vi "MegaAnalysis5.vi"() -> ()   [LabVIEW 2016] (continued)
                      n495 = call <vilib>:"Check if File or Folder Exists.vi"("path"=w1236) -> ("file or folder exists?"=w1237:bool)  [unwired: 1 in, 9 out]
                      n496 = case shown="True" w1237 {
                        selector: w1237 -> [_ w1239]
                        tunnel: w1236 -> [_ w1238]
                        frame False {
                        }
                        frame True {
                          n497 = Delete(path (use dialog)=w1238, entire hierarchy (F)=w1239) -> ()  [unwired: 1 in, 5 out]
                        }
                      }
                    }
                    frame #1 {
                      n498 = Write to Text File(file (use dialog)=w1240, text=w1241) -> ()  [unwired: 1 in, 4 out]
                    }
                    frame #2 {
                      w1242 = TRUE
                      n499 = call "Write To Spreadsheet File2.vi"("transpose? (no:F)"=w1242, "format (%d)"=w1243, "append to file? (new file:F)"=w1242, "2D data"=w1245, "file path (dialog if empty)"=w1244) -> ()  [unwired: 3 in, 1 out]
                    }
                  }
                }
                n500 = global write "status.vi" "String"("saving import") -> ()
              }
            }
          }
          frame #19 {
            n501 = Or(x=w1254, y="?") -> (x .or. y?=w1255:bool)
            n502 = Reciprocal(x=w1258) -> (1/x=w1264:ext[])
            "sampling frequency" <- w1264
            n503 = Not Equal To 0?(x=w1258) -> (x != 0?=w1265:bool[])
            n504 = for {
              tunnel: w1255 -> [w1277]
              tunnel: "filter selection" -> [w1278]
              tunnel: w1265 -> [w1276] mode=indexing
              tunnel: w1264 -> [w1275] mode=indexing
              tunnel: w1263 -> [w1272]
              tunnel: "high cutoff freq: fh" -> [w1271]
              tunnel: "low cutoff freq: fl" -> [w1270]
              tunnel: "filter type" -> [w1269]
              tunnel: "order" -> [w1268]
              tunnel: w1257 -> [w1267]
              i -> [w1273]
              n505 = And(x=w1277, y=w1276) -> (x .and. y?=w1274:bool)
              n506 = case shown="True" w1274 {
                tunnel: w1278 -> [_ w1288]
                tunnel: w1275 -> [_ w1287]
                tunnel: w1273 -> [_ w1286]
                tunnel: w1272 -> [_ w1285]
                tunnel: w1271 -> [_ w1284]
                tunnel: w1270 -> [_ w1283]
                tunnel: w1269 -> [_ w1282]
                tunnel: w1268 -> [_ w1281]
                tunnel: w1267 -> [_ w1280]
                frame False {
                }
                frame True {
                  n507 = case shown="0, Default" w1288 {
                    tunnel: w1287 -> [_ w1294 w1309 w1324 w1340 w1354 w1370 _]
                    tunnel: w1286 -> [_ w1300 w1316 w1331 w1347 w1361 w1366 w1385]
                    tunnel: w1285 -> [_ w1299 w1315 w1330 w1346 w1360 w1376 w1387]
                    tunnel: w1284 -> [_ w1293 w1308 w1323 w1339 w1353 w1368 _]
                    tunnel: w1283 -> [_ w1292 w1307 w1322 w1338 w1352 w1369 _]
                    tunnel: w1282 -> [_ w1291 w1304 w1321 w1337 w1350 w1367 _]
                    tunnel: w1281 -> [_ w1290 w1306 w1319 w1336 w1351 _ _]
                    tunnel: w1280 -> [_ w1289 w1303 w1318 w1333 w1349 w1363 w1378]
                    frame 0, Default {
                    }
                    frame 1 {
                      w1301 = "dat2"
                      w1302 = "dat1"
                      n508 = call "readbinary.vi"(7:w1289, "base path"=w1299, "file index"=w1300, "data column"=w1302) -> ("data"=w1297:ext[])  [unwired: 7 out]
                      n509 = call "readbinary.vi"(7:w1289, "base path"=w1299, "file index"=w1300, "data column"=w1301) -> ("data"=w1298:ext[])  [unwired: 7 out]
                      n510 = call-poly <vilib>:"Butterworth Filter.vi"("order"=w1290, "filter type"=w1291, "low cutoff freq: fl"=w1292, "high cutoff freq: fh"=w1293, "sampling freq: fs"=w1294, "X"=w1297) -> ("Filtered X"=w1296:dbl[])  [unwired: 1 in, 2 out]
                      n511 = call-poly <vilib>:"Butterworth Filter.vi"("order"=w1290, "filter type"=w1291, "low cutoff freq: fl"=w1292, "high cutoff freq: fh"=w1293, "sampling freq: fs"=w1294, "X"=w1298) -> ("Filtered X"=w1295:dbl[])  [unwired: 1 in, 2 out]
                      n512 = call "writebinary.vi"(7:w1289, "base path"=w1299, "file index"=w1300, "data column"=w1302, "data"=w1296) -> ()  [unwired: 7 out]
                      n513 = call "writebinary.vi"(7:w1289, "base path"=w1299, "file index"=w1300, "data column"=w1301, "data"=w1295) -> ()  [unwired: 7 out]
                    }
                    frame 2 {
                      w1317 = "dat2"
                      w1313 = "dat1"
                      n514 = call "readbinary.vi"(7:w1303, "base path"=w1315, "file index"=w1316, "data column"=w1313) -> ("data"=w1312:ext[])  [unwired: 7 out]
                      n515 = call "readbinary.vi"(7:w1303, "base path"=w1315, "file index"=w1316, "data column"=w1317) -> ("data"=w1314:ext[])  [unwired: 7 out]
                      n516 = call-poly <vilib>:"Chebyshev Filter.vi"("order"=w1306, "ripple(dB)"="ripple(dB)", "filter type"=w1304, "low cutoff freq: fl"=w1307, "high cutoff freq: fh"=w1308, "sampling freq: fs"=w1309, "X"=w1314) -> ("Filtered X"=w1310:dbl[])  [unwired: 1 in, 3 out]
                      n517 = call-poly <vilib>:"Chebyshev Filter.vi"("order"=w1306, "ripple(dB)"="ripple(dB)", "filter type"=w1304, "low cutoff freq: fl"=w1307, "high cutoff freq: fh"=w1308, "sampling freq: fs"=w1309, "X"=w1312) -> ("Filtered X"=w1311:dbl[])  [unwired: 1 in, 3 out]
                      n518 = call "writebinary.vi"(7:w1303, "base path"=w1315, "file index"=w1316, "data column"=w1313, "data"=w1311) -> ()  [unwired: 7 out]
                      n519 = call "writebinary.vi"(7:w1303, "base path"=w1315, "file index"=w1316, "data column"=w1317, "data"=w1310) -> ()  [unwired: 7 out]
                    }
                    frame 3 {
                      w1332 = "dat2"
                      w1329 = "dat1"
                      n520 = call "readbinary.vi"(7:w1318, "base path"=w1330, "file index"=w1331, "data column"=w1329) -> ("data"=w1326:ext[])  [unwired: 7 out]
                      n521 = call "readbinary.vi"(7:w1318, "base path"=w1330, "file index"=w1331, "data column"=w1332) -> ("data"=w1328:ext[])  [unwired: 7 out]
                      n522 = call-poly <vilib>:"Inverse Chebyshev Filter.vi"("order"=w1319, "attenuation (dB)"="attenuation (dB)", "filter type"=w1321, "low cutoff freq: fl"=w1322, "high cutoff freq: fh"=w1323, "sampling freq: fs"=w1324, "X"=w1328) -> ("Filtered X"=w1327:dbl[])  [unwired: 1 in, 3 out]
                      n523 = call-poly <vilib>:"Inverse Chebyshev Filter.vi"("order"=w1319, "attenuation (dB)"="attenuation (dB)", "filter type"=w1321, "low cutoff freq: fl"=w1322, "high cutoff freq: fh"=w1323, "sampling freq: fs"=w1324, "X"=w1326) -> ("Filtered X"=w1325:dbl[])  [unwired: 1 in, 3 out]
                      n524 = call "writebinary.vi"(7:w1318, "base path"=w1330, "file index"=w1331, "data column"=w1329, "data"=w1325) -> ()  [unwired: 7 out]
                      n525 = call "writebinary.vi"(7:w1318, "base path"=w1330, "file index"=w1331, "data column"=w1332, "data"=w1327) -> ()  [unwired: 7 out]
                    }
                    frame 4 {
                      w1348 = "dat2"
                      w1345 = "dat1"
                      n526 = call "readbinary.vi"(7:w1333, "base path"=w1346, "file index"=w1347, "data column"=w1345) -> ("data"=w1343:ext[])  [unwired: 7 out]
                      n527 = call "readbinary.vi"(7:w1333, "base path"=w1346, "file index"=w1347, "data column"=w1348) -> ("data"=w1344:ext[])  [unwired: 7 out]
                      n528 = call-poly <vilib>:"Elliptic Filter.vi"("order"=w1336, "filter type"=w1337, "stopband attenuation (dB)"="stopband attenuation (dB)", "passband ripple (dB)"="passband ripple (dB)", "low cutoff freq: fl"=w1338, "high cutoff freq: fh"=w1339, "sampling freq: fs"=w1340, "X"=w1343) -> ("Filtered X"=w1342:dbl[])  [unwired: 1 in, 2 out]
                      n529 = call-poly <vilib>:"Elliptic Filter.vi"("order"=w1336, "filter type"=w1337, "stopband attenuation (dB)"="stopband attenuation (dB)", "passband ripple (dB)"="passband ripple (dB)", "low cutoff freq: fl"=w1338, "high cutoff freq: fh"=w1339, "sampling freq: fs"=w1340, "X"=w1344) -> ("Filtered X"=w1341:dbl[])  [unwired: 1 in, 2 out]
                      n530 = call "writebinary.vi"(7:w1333, "base path"=w1346, "file index"=w1347, "data column"=w1345, "data"=w1342) -> ()  [unwired: 7 out]
                      n531 = call "writebinary.vi"(7:w1333, "base path"=w1346, "file index"=w1347, "data column"=w1348, "data"=w1341) -> ()  [unwired: 7 out]
                    }
                    frame 5 {
                      w1362 = "dat2"
                      w1359 = "dat1"
                      n532 = call "readbinary.vi"(7:w1349, "base path"=w1360, "file index"=w1361, "data column"=w1359) -> ("data"=w1357:ext[])  [unwired: 7 out]
                      n533 = call "readbinary.vi"(7:w1349, "base path"=w1360, "file index"=w1361, "data column"=w1362) -> ("data"=w1358:ext[])  [unwired: 7 out]
                      n534 = call-poly <vilib>:"Bessel Filter.vi"("order"=w1351, "filter type"=w1350, "low cutoff freq: fl"=w1352, "high cutoff freq: fh"=w1353, "sampling freq: fs"=w1354, "X"=w1357) -> ("Filtered X"=w1356:dbl[])  [unwired: 1 in, 2 out]
                      n535 = call-poly <vilib>:"Bessel Filter.vi"("order"=w1351, "filter type"=w1350, "low cutoff freq: fl"=w1352, "high cutoff freq: fh"=w1353, "sampling freq: fs"=w1354, "X"=w1358) -> ("Filtered X"=w1355:dbl[])  [unwired: 1 in, 2 out]
                      n536 = call "writebinary.vi"(7:w1349, "base path"=w1360, "file index"=w1361, "data column"=w1359, "data"=w1356) -> ()  [unwired: 7 out]
                      n537 = call "writebinary.vi"(7:w1349, "base path"=w1360, "file index"=w1361, "data column"=w1362, "data"=w1355) -> ()  [unwired: 7 out]
                    }
                    frame 6 {
                      w1377 = "dat2"
                      w1375 = "dat1"
                      n538 = call "readbinary.vi"(7:w1363, "base path"=w1376, "file index"=w1366, "data column"=w1375) -> ("data"=w1373:ext[])  [unwired: 7 out]
                      n539 = call "readbinary.vi"(7:w1363, "base path"=w1376, "file index"=w1366, "data column"=w1377) -> ("data"=w1374:ext[])  [unwired: 7 out]
                      n540 = call <vilib>:"FIR Windowed Filter (obs).vi"("sampling freq: fs"=w1370, "X"=w1373, "filter type"=w1367, "low cutoff freq: fl"=w1369, "high cutoff freq: fh"=w1368, "taps"="taps", "window"="window") -> ("Filtered X"=w1372:dbl[])  [unwired: 8 out]
                      n541 = call <vilib>:"FIR Windowed Filter (obs).vi"("sampling freq: fs"=w1370, "X"=w1374, "filter type"=w1367, "low cutoff freq: fl"=w1369, "high cutoff freq: fh"=w1368, "taps"="taps", "window"="window") -> ("Filtered X"=w1371:dbl[])  [unwired: 8 out]
                      n542 = call "writebinary.vi"(7:w1363, "base path"=w1376, "file index"=w1366, "data column"=w1375, "data"=w1372) -> ()  [unwired: 7 out]
                      n543 = call "writebinary.vi"(7:w1363, "base path"=w1376, "file index"=w1366, "data column"=w1377, "data"=w1371) -> ()  [unwired: 7 out]
                    }
                    frame 7 {
                      w1388 = "dat2"
                      w1386 = "dat1"
                      n544 = call "readbinary.vi"(7:w1378, "base path"=w1387, "file index"=w1385, "data column"=w1386) -> ("data"=w1383:ext[])  [unwired: 7 out]
                      n545 = call "readbinary.vi"(7:w1378, "base path"=w1387, "file index"=w1385, "data column"=w1388) -> ("data"=w1384:ext[])  [unwired: 7 out]
                      n546 = call <vilib>:"Median Filter.vi"("right rank"="right rank", "left rank"="left rank", "X"=w1383) -> ("Filtered X"=w1382:dbl[])  [unwired: 8 out]
                      n547 = call <vilib>:"Median Filter.vi"("right rank"="right rank", "left rank"="left rank", "X"=w1384) -> ("Filtered X"=w1381:dbl[])  [unwired: 8 out]
                      n548 = call "writebinary.vi"(7:w1378, "base path"=w1387, "file index"=w1385, "data column"=w1386, "data"=w1382) -> ()  [unwired: 7 out]
                      n549 = call "writebinary.vi"(7:w1378, "base path"=w1387, "file index"=w1385, "data column"=w1388, "data"=w1381) -> ()  [unwired: 7 out]
                    }
                  }
                  n550 = global write "status.vi" "String"("filtering") -> ()
                }
              }
            }
          }
          frame #20 {
            n551 = case shown="True" w1392 {
              tunnel: w1391 -> [_ w1395]
              tunnel: w1390 -> [_ w1394]
              tunnel: w1389 -> [_ w1393]
              frame False {
              }
              frame True {
                n552 = Path To String(path=w1394) -> (string=w1400:string[])
                n553 = Build Path(base path=w1395, name or relative path="files") -> (appended path=w1397:path)
                n554 = call-poly <vilib>:"Write To Spreadsheet File.vi"("1D data"=w1393, "file path (dialog if empty)"=w1397) -> ()  [unwired: 4 in, 3 out]
                n555 = Build Path(base path=w1395, name or relative path="paths") -> (appended path=w1399:path)
                n556 = call-poly <vilib>:"Write To Spreadsheet File.vi"("1D data"=w1400, "file path (dialog if empty)"=w1399) -> ()  [unwired: 4 in, 3 out]
              }
            }
          }
        }
      }
      frame #5 {
        # "select frame"
        # "old"
        # "both"
        # "rising"
        # "falling"
        # "c"
        # "p"
        n557 = Equal?(x=w1416, y=2) -> (x = y?=w1412:bool)
        n558 = Equal?(x="?", y=5) -> (x = y?=w1411:bool)
        n559 = And(x=w1412, y=w1411) -> (x .and. y?=w1410:bool)
        n560 = Or(x="?", y=w1403) -> (x .or. y?=w1405:bool)
        n561 = stacked-sequence {
          seq-local: [w1435 _ _ _ _ _ _ _ _ _] -> [_ _ _ _ _ w2421 w2652 w3048 w3122 _]
          seq-local: [w1434 _ _ _ _ _ _ _ _ _] -> [_ _ _ _ _ w2420 w2651 w3049 w3113 _]
          seq-local: [w1433 _ _ _ _ _ _ _ _ _] -> [_ w1485 w2161 _ _ w2422 _ _ _ _]
          seq-local: [w1422 _ _ _ _ _ _ _ _ _] -> [_ w1484 _ _ _ _ _ _ _ _]
          tunnel: w1405 -> [_ w1486 w2160 w2233 w2389 w2424 w2654 _ _ _]
          tunnel: w1417 -> [w1418 w1489 w2162 w2232 w2388 w2423 w2653 w3050 w3112 w3202]
          tunnel: w1410 -> [_ _ _ _ _ _ _ w3051 _ _]
          tunnel: "?" -> [_ _ _ _ _ _ _ _ w3123 _]
          tunnel: w1408 -> [_ w1483 _ _ _ _ _ _ w3111 _]
          tunnel: w1407 -> [w1419 w1482 w2159 w2231 w2387 w2419 w2650 w3046 _ _]
          tunnel: w1406 -> [w1420 _ _ _ _ _ _ _ _ _]
          tunnel: w1402 -> [_ _ _ _ _ _ _ _ w3110 _]
          tunnel: [_ _ _ _ _ _ _ _ w3109 _] -> w1401
          frame #0 {
            n562 = Build Array("indr", "timr", "bdtr", "bclr", "datr") -> (w1435:string[])
            n563 = Build Array("indf", "timf", "bdtf", "bclf", "datf") -> (w1434:string[])
            n564 = Build Array("indx", "time", "bdot", "bcol", "dat1", "dat2") -> (w1422:string[])
            n565 = Build Array("indt", "timt", "bdtt", "bclt", "dt1t", "dt2t") -> (w1433:string[])
            n566 = Build Path(base path=w1418, name or relative path="files") -> (appended path=w1430:path)
            n567 = Build Array (concatenate)(w1435, w1434, w1433) -> (w1432:string[])
            n568 = call-poly <vilib>:"Read From Spreadsheet File.vi"("file path (dialog if empty)"=w1430) -> ("first row"=w1429:string[])  [unwired: 3 in, 7 out]
            n569 = stacked-sequence {
              tunnel: w1432 -> [w1453 w1465]
              tunnel: w1418 -> [w1452 w1464]
              tunnel: w1429 -> [w1451 w1463]
              tunnel: w1420 -> [_ w1461]
              tunnel: w1419 -> [_ w1460]
              frame #0 {
                n570 = for {
                  tunnel: w1453 -> [w1456]
                  tunnel: w1452 -> [w1455]
                  tunnel: w1451 -> [_] mode=indexing
                  i -> [w1454]
                  n571 = for {
                    tunnel: w1456 -> [w1459] mode=indexing
                    tunnel: w1455 -> [w1458]
                    tunnel: w1454 -> [w1457]
                    n572 = call "createemptybinary.vi"("base path"=w1458, "file index"=w1457, "data column"=w1459) -> ()  [unwired: 9 out]
                  }
                }
              }
              frame #1 {
                n573 = Equal?(x=w1461, y=w1460) -> (x = y?=w1462:bool)
                n574 = case shown="False" w1462 {
                  tunnel: w1463 -> [w1470 _]
                  tunnel: w1465 -> [w1469 _]
                  tunnel: w1461 -> [w1468 _]
                  tunnel: w1460 -> [w1467 _]
                  tunnel: w1464 -> [w1466 _]
                  frame False {
                    n575 = for {
                      tunnel: w1470 -> [_] mode=indexing
                      tunnel: w1469 -> [w1475]
                      tunnel: w1466 -> [w1473]
                      tunnel: w1468 -> [w1472]
                      tunnel: w1467 -> [w1471]
                      i -> [w1474]
                      n576 = for {
                        tunnel: w1475 -> [w1478] mode=indexing
                        tunnel: w1474 -> [w1477]
                        tunnel: w1473 -> [w1476]
                        tunnel: w1472 -> [w1481]
                        tunnel: w1471 -> [w1479]
                        n577 = call "readbinary.vi"(7:w1481, "base path"=w1476, "file index"=w1477, "data column"=w1478) -> ("data"=w1480:ext[])  [unwired: 7 out]
                        n578 = call "writebinary.vi"(7:w1479, "base path"=w1476, "file index"=w1477, "data column"=w1478, "data"=w1480) -> ()  [unwired: 7 out]
                      }
                    }
                  }
                  frame True {
                  }
                }
              }
            }
          }
          frame #1 {
            n579 = case shown="False" w1486 {
              tunnel: "?" -> [_ w1501]
              tunnel: "reference option" -> [_ w1500]
              tunnel: w1489 -> [_ w1499]
              tunnel: "file name options" -> [_ w1498]
              tunnel: "?" -> [_ w1497]
              tunnel: w1485 -> [_ w1496]
              tunnel: w1484 -> [_ w1495]
              tunnel: w1483 -> [_ w1494]
              tunnel: w1482 -> [_ w1493]
              frame False {
              }
              frame True {
                n580 = case shown="False" w1501 {
                  tunnel: w1500 -> [_ w1536]
                  tunnel: w1499 -> [w1505 w1535]
                  tunnel: w1498 -> [_ w1534]
                  tunnel: w1497 -> [_ w1533]
                  tunnel: w1496 -> [w1506 _]
                  tunnel: w1495 -> [w1504 _]
                  tunnel: w1494 -> [w1503 w1532]
                  tunnel: w1493 -> [w1502 w1531]
                  frame False {
                    n581 = Build Path(base path=w1505, name or relative path="paths") -> (appended path=w1513:path)
                    n582 = Build Path(base path=w1505, name or relative path="files") -> (appended path=w1514:path)
                    n583 = call-poly <vilib>:"Read From Spreadsheet File.vi"("file path (dialog if empty)"=w1513) -> ("first row"=w1507:string[])  [unwired: 3 in, 7 out]
                    n584 = call-poly <vilib>:"Read From Spreadsheet File.vi"("file path (dialog if empty)"=w1514) -> ("first row"=w1508:string[])  [unwired: 3 in, 7 out]
                    n585 = Build Path(base path=w1505, name or relative path="files2") -> (appended path=w1510:path)
                    n586 = Build Path(base path=w1505, name or relative path="paths2") -> (appended path=w1509:path)
                    n587 = for {
                      tunnel: w1507 -> [_] mode=indexing
                      tunnel: w1506 -> [w1522]
                      tunnel: w1505 -> [w1521]
                      tunnel: w1504 -> [w1520]
                      tunnel: w1503 -> [w1518]
                      tunnel: w1502 -> [w1517]
                      i -> [w1519]
                      n588 = for {
                        tunnel: w1522 -> [w1527] mode=indexing
                        tunnel: w1519 -> [w1530]
                        tunnel: w1521 -> [w1525]
                        tunnel: w1520 -> [w1529] mode=indexing
                        tunnel: w1519 -> [w1526]
                        tunnel: w1518 -> [w1524]
                        tunnel: w1517 -> [w1523]
                        n589 = call "readbinary.vi"(7:w1524, "base path"=w1525, "file index"=w1530, "data column"=w1529) -> ("data"=w1528:ext[])  [unwired: 7 out]
                        n590 = call "writebinary.vi"(7:w1523, "base path"=w1525, "file index"=w1526, "data column"=w1527, "data"=w1528) -> ()  [unwired: 7 out]
                      }
                    }
                    n591 = call-poly <vilib>:"Write To Spreadsheet File.vi"("1D data"=w1508, "file path (dialog if empty)"=w1510) -> ()  [unwired: 4 in, 3 out]
                    n592 = call-poly <vilib>:"Write To Spreadsheet File.vi"("1D data"=w1507, "file path (dialog if empty)"=w1509) -> ()  [unwired: 4 in, 3 out]
                  }
                  frame True {
                    n593 = case shown="1" w1536 {
                      tunnel: w1535 -> [w1541 w1701 w1851 w2011]
                      tunnel: w1534 -> [w1540 w1700 w1850 w2010]
                      tunnel: w1533 -> [w1539 w1699 w1849 w2009]
                      tunnel: w1532 -> [w1538 w1698 w1848 w2008]
                      tunnel: w1531 -> [w1537 w1697 w1847 w2007]
                      frame 0, Default {
                        n594 = stacked-sequence {
                          seq-local: [w1544 _ _ _ _ _ _ _] -> [_ w1557 w1576 w1595 w1616 w1637 w1653 w1674]
                          seq-local: [w1542 _ _ _ _ _ _ _] -> [_ _ _ _ _ _ _ w1671]
                          tunnel: w1541 -> [w1548 w1553 w1572 w1591 w1612 w1633 w1649 w1663]
                          tunnel: w1540 -> [_ _ _ _ _ _ _ w1673]
                          tunnel: w1539 -> [_ _ _ _ _ _ _ w1672]
                          tunnel: w1538 -> [_ w1552 w1571 w1590 w1611 w1632 w1648 _]
                          tunnel: w1537 -> [_ w1551 w1570 w1589 w1610 w1631 w1647 _]
                          frame #0 {
                            w1546 = "%s"
                            n595 = Build Path(base path=w1548, name or relative path="files") -> (appended path=w1549:path)
                            n596 = call-poly <vilib>:"Read From Spreadsheet File.vi"("format (%s)"=w1546, "file path (dialog if empty)"=w1549) -> ("first row"=w1544:string[])  [unwired: 2 in, 7 out]
                            n597 = Build Path(base path=w1548, name or relative path="paths") -> (appended path=w1545:path)
                            n598 = call-poly <vilib>:"Read From Spreadsheet File.vi"("format (%s)"=w1546, "file path (dialog if empty)"=w1545) -> ("first row"=w1543:string[])  [unwired: 2 in, 7 out]
                            n599 = String To Path(string=w1543) -> (path=w1542:path[])
                          }
                          frame #1 {
                            n600 = Array Size(array=w1557) -> (size(s)=w1556:i32)
                            n601 = Divide(x=w1556, y=2) -> (x/y=w1554:dbl)
                            n602 = for {
                              N: w1554 -> [_]
                              tunnel: w1553 -> [w1561]
                              tunnel: w1552 -> [w1559]
                              tunnel: w1551 -> [w1558]
                              i -> [w1562]
                              w1564 = "dat1"
                              n603 = Multiply(x=2, y=w1562) -> (x*y=w1568:i32)
                              n604 = Increment(x=w1568) -> (x+1=w1567:i32)
                              n605 = call "readbinary.vi"(7:w1559, "base path"=w1561, "file index"=w1568, "data column"=w1564) -> ("data"=w1566:ext[])  [unwired: 7 out]
                              n606 = call "readbinary.vi"(7:w1559, "base path"=w1561, "file index"=w1567, "data column"=w1564) -> ("data"=w1565:ext[])  [unwired: 7 out]
                              n607 = Subtract(x=w1566, y=w1565) -> (x-y=w1563:ext[])
                              n608 = call "writebinary.vi"(7:w1558, "base path"=w1561, "file index"=w1562, "data column"="dt1t", "data"=w1563) -> ()  [unwired: 7 out]
                            }
                          }
                          frame #2 {
                            n609 = Array Size(array=w1576) -> (size(s)=w1575:i32)
                            n610 = Divide(x=w1575, y=2) -> (x/y=w1573:dbl)
                            n611 = for {
                              N: w1573 -> [_]
                              tunnel: w1572 -> [w1580]
                              tunnel: w1571 -> [w1578]
                              tunnel: w1570 -> [w1577]
                              i -> [w1581]
                              w1583 = "dat2"
                              n612 = Multiply(x=2, y=w1581) -> (x*y=w1587:i32)
                              n613 = Increment(x=w1587) -> (x+1=w1586:i32)
                              n614 = call "readbinary.vi"(7:w1578, "base path"=w1580, "file index"=w1587, "data column"=w1583) -> ("data"=w1585:ext[])  [unwired: 7 out]
                              n615 = call "readbinary.vi"(7:w1578, "base path"=w1580, "file index"=w1586, "data column"=w1583) -> ("data"=w1584:ext[])  [unwired: 7 out]
                              n616 = Subtract(x=w1585, y=w1584) -> (x-y=w1582:ext[])
                              n617 = call "writebinary.vi"(7:w1577, "base path"=w1580, "file index"=w1581, "data column"="dt2t", "data"=w1582) -> ()  [unwired: 7 out]
                            }
                          }
                          frame #3 {
                            n618 = Array Size(array=w1595) -> (size(s)=w1594:i32)
                            n619 = Divide(x=w1594, y=2) -> (x/y=w1592:dbl)
                            n620 = for {
                              N: w1592 -> [_]
                              tunnel: w1591 -> [w1604]
                              tunnel: w1590 -> [w1597]
                              tunnel: w1589 -> [w1596]
                              i -> [w1605]
                              w1606 = "bcol"
                              n621 = Multiply(x=2, y=w1605) -> (x*y=w1608:i32)
                              n622 = Increment(x=w1608) -> (x+1=w1607:i32)
                              n623 = call "readbinary.vi"(7:w1597, "base path"=w1604, "file index"=w1608, "data column"=w1606) -> ("data"=w1601:ext[])  [unwired: 7 out]
                              n624 = call "readbinary.vi"(7:w1597, "base path"=w1604, "file index"=w1607, "data column"=w1606) -> ("data"=w1600:ext[])  [unwired: 7 out]
                              n625 = Add(x=w1601, y=w1600) -> (x+y=w1603:ext[])
                              n626 = Divide(x=w1603, y=2) -> (x/y=w1599:ext[])
                              n627 = call "writebinary.vi"(7:w1596, "base path"=w1604, "file index"=w1605, "data column"="bclt", "data"=w1599) -> ()  [unwired: 7 out]
                            }
                          }
                          frame #4 {
                            n628 = Array Size(array=w1616) -> (size(s)=w1615:i32)
                            n629 = Divide(x=w1615, y=2) -> (x/y=w1613:dbl)
                            n630 = for {
                              N: w1613 -> [_]
                              tunnel: w1612 -> [w1625]
                              tunnel: w1611 -> [w1618]
                              tunnel: w1610 -> [w1617]
                              i -> [w1626]
                              w1627 = "bdot"
                              n631 = Multiply(x=2, y=w1626) -> (x*y=w1629:i32)
                              n632 = Increment(x=w1629) -> (x+1=w1628:i32)
                              n633 = call "readbinary.vi"(7:w1618, "base path"=w1625, "file index"=w1629, "data column"=w1627) -> ("data"=w1622:ext[])  [unwired: 7 out]
                              n634 = call "readbinary.vi"(7:w1618, "base path"=w1625, "file index"=w1628, "data column"=w1627) -> ("data"=w1621:ext[])  [unwired: 7 out]
                              n635 = Add(x=w1622, y=w1621) -> (x+y=w1624:ext[])
                              n636 = Divide(x=w1624, y=2) -> (x/y=w1620:ext[])
                              n637 = call "writebinary.vi"(7:w1617, "base path"=w1625, "file index"=w1626, "data column"="bdtt", "data"=w1620) -> ()  [unwired: 7 out]
                            }
                          }
                          frame #5 {
                            n638 = Array Size(array=w1637) -> (size(s)=w1636:i32)
                            n639 = Divide(x=w1636, y=2) -> (x/y=w1634:dbl)
                            n640 = for {
                              N: w1634 -> [_]
                              tunnel: w1633 -> [w1642]
                              tunnel: w1632 -> [w1639]
                              tunnel: w1631 -> [w1638]
                              i -> [w1643]
                              n641 = Multiply(x=2, y=w1643) -> (x*y=w1645:i32)
                              n642 = Increment(x=w1645) -> ()  [unwired: 1 out]
                              n643 = call "readbinary.vi"(7:w1639, "base path"=w1642, "file index"=w1645, "data column"="indx") -> ("data"=w1641:ext[])  [unwired: 7 out]
                              n644 = call "writebinary.vi"(7:w1638, "base path"=w1642, "file index"=w1643, "data column"="indt", "data"=w1641) -> ()  [unwired: 7 out]
                            }
                          }
                          frame #6 {
                            n645 = Array Size(array=w1653) -> (size(s)=w1652:i32)
                            n646 = Divide(x=w1652, y=2) -> (x/y=w1650:dbl)
                            n647 = for {
                              N: w1650 -> [_]
                              tunnel: w1649 -> [w1658]
                              tunnel: w1648 -> [w1655]
                              tunnel: w1647 -> [w1654]
                              i -> [w1659]
                              n648 = Multiply(x=2, y=w1659) -> (x*y=w1661:i32)
                              n649 = Increment(x=w1661) -> ()  [unwired: 1 out]
                              n650 = call "readbinary.vi"(7:w1655, "base path"=w1658, "file index"=w1661, "data column"="time") -> ("data"=w1657:ext[])  [unwired: 7 out]
                              n651 = call "writebinary.vi"(7:w1654, "base path"=w1658, "file index"=w1659, "data column"="timt", "data"=w1657) -> ()  [unwired: 7 out]
                            }
                          }
                          frame #7 {
                            n652 = Array Size(array=w1674) -> (size(s)=w1677:i32)
                            n653 = Divide(x=w1677, y=2) -> (x/y=w1675:dbl)
                            n654 = for {
                              N: w1675 -> [_]
                              tunnel: w1663 -> [_]
                              tunnel: w1674 -> [w1686]
                              tunnel: w1673 -> [w1685]
                              tunnel: w1672 -> [w1682]
                              tunnel: [w1681] -> w1665 mode=indexing
                              tunnel: w1671 -> [w1680]
                              tunnel: [w1678] -> w1666 mode=indexing
                              i -> [w1688]
                              n655 = Multiply(x=2, y=w1688) -> (x*y=w1679:i32)
                              n656 = Index Array(array=w1686, index=w1679) -> (element=w1684:string)
                              n657 = Increment(x=w1679) -> (x+1=w1687:i32)
                              n658 = Index Array(array=w1686, index=w1687) -> (element=w1683:string)
                              n659 = case shown="1" w1685 {
                                tunnel: w1684 -> [w1690 w1696]
                                tunnel: w1683 -> [_ w1695]
                                tunnel: [w1690 w1693] -> w1681
                                tunnel: w1682 -> [_ w1694]
                                frame 0, Default {
                                }
                                frame 1 {
                                n660 = String Subset(string=w1696, length (rest)=w1694) -> (substring=w1692:string)  [unwired: 1 out]
                                n661 = String Subset(string=w1695, length (rest)=w1694) -> (substring=w1691:string)  [unwired: 1 out]
                                n662 = Concatenate Strings(w1692, w1691) -> (w1693:string)
                                }
                              }
                              n663 = Index Array(array=w1680, index=w1679) -> (element=w1678:path)
                            }
                            n664 = Build Path(base path=w1663, name or relative path="files2") -> (appended path=w1669:path)
                            n665 = call-poly <vilib>:"Write To Spreadsheet File.vi"("1D data"=w1665, "file path (dialog if empty)"=w1669) -> ()  [unwired: 4 in, 3 out]
                            n666 = Build Path(base path=w1663, name or relative path="paths2") -> (appended path=w1667:path)
                            n667 = Path To String(path=w1666) -> (string=w1664:string[])
                            n668 = call-poly <vilib>:"Write To Spreadsheet File.vi"("1D data"=w1664, "file path (dialog if empty)"=w1667) -> ()  [unwired: 4 in, 3 out]
                          }
                        }
                      }
                      frame 2 {
                        n669 = stacked-sequence {
                          seq-local: [w1704 _ _ _ _ _ _ _] -> [_ w1717 w1736 w1755 w1771 w1787 w1803 w1824]
                          seq-local: [w1702 _ _ _ _ _ _ _] -> [_ _ _ _ _ _ _ w1821]
                          tunnel: w1701 -> [w1708 w1713 w1732 w1751 w1767 w1783 w1799 w1813]
                          tunnel: w1700 -> [_ _ _ _ _ _ _ w1823]
                          tunnel: w1699 -> [_ _ _ _ _ _ _ w1822]
                          tunnel: w1698 -> [_ w1712 w1731 w1750 w1766 w1782 w1798 _]
                          tunnel: w1697 -> [_ w1711 w1730 w1749 w1765 w1781 w1797 _]
                          frame #0 {
                            w1706 = "%s"
                            n670 = Build Path(base path=w1708, name or relative path="files") -> (appended path=w1709:path)
                            n671 = call-poly <vilib>:"Read From Spreadsheet File.vi"("format (%s)"=w1706, "file path (dialog if empty)"=w1709) -> ("first row"=w1704:string[])  [unwired: 2 in, 7 out]
                            n672 = Build Path(base path=w1708, name or relative path="paths") -> (appended path=w1705:path)
                            n673 = call-poly <vilib>:"Read From Spreadsheet File.vi"("format (%s)"=w1706, "file path (dialog if empty)"=w1705) -> ("first row"=w1703:string[])  [unwired: 2 in, 7 out]
                            n674 = String To Path(string=w1703) -> (path=w1702:path[])
                          }
                          frame #1 {
                            n675 = Array Size(array=w1717) -> (size(s)=w1716:i32)
                            n676 = Divide(x=w1716, y=2) -> (x/y=w1714:dbl)
                            n677 = for {
                              N: w1714 -> [_]
                              tunnel: w1713 -> [w1721]
                              tunnel: w1712 -> [w1719]
                              tunnel: w1711 -> [w1718]
                              i -> [w1722]
                              w1724 = "dat1"
                              n678 = Multiply(x=2, y=w1722) -> (x*y=w1728:i32)
                              n679 = Increment(x=w1728) -> (x+1=w1727:i32)
                              n680 = call "readbinary.vi"(7:w1719, "base path"=w1721, "file index"=w1728, "data column"=w1724) -> ("data"=w1726:ext[])  [unwired: 7 out]
                              n681 = call "readbinary.vi"(7:w1719, "base path"=w1721, "file index"=w1727, "data column"=w1724) -> ("data"=w1725:ext[])  [unwired: 7 out]
                              n682 = Subtract(x=w1726, y=w1725) -> (x-y=w1723:ext[])
                              n683 = call "writebinary.vi"(7:w1718, "base path"=w1721, "file index"=w1722, "data column"="dt1t", "data"=w1723) -> ()  [unwired: 7 out]
                            }
                          }
                          frame #2 {
                            n684 = Array Size(array=w1736) -> (size(s)=w1735:i32)
                            n685 = Divide(x=w1735, y=2) -> (x/y=w1733:dbl)
                            n686 = for {
                              N: w1733 -> [_]
                              tunnel: w1732 -> [w1740]
                              tunnel: w1731 -> [w1738]
                              tunnel: w1730 -> [w1737]
                              i -> [w1741]
                              w1743 = "dat2"
                              n687 = Multiply(x=2, y=w1741) -> (x*y=w1747:i32)
                              n688 = Increment(x=w1747) -> (x+1=w1746:i32)
                              n689 = call "readbinary.vi"(7:w1738, "base path"=w1740, "file index"=w1747, "data column"=w1743) -> ("data"=w1745:ext[])  [unwired: 7 out]
                              n690 = call "readbinary.vi"(7:w1738, "base path"=w1740, "file index"=w1746, "data column"=w1743) -> ("data"=w1744:ext[])  [unwired: 7 out]
                              n691 = Subtract(x=w1745, y=w1744) -> (x-y=w1742:ext[])
                              n692 = call "writebinary.vi"(7:w1737, "base path"=w1740, "file index"=w1741, "data column"="dt2t", "data"=w1742) -> ()  [unwired: 7 out]
                            }
                          }
                          frame #3 {
                            n693 = Array Size(array=w1755) -> (size(s)=w1754:i32)
                            n694 = Divide(x=w1754, y=2) -> (x/y=w1752:dbl)
                            n695 = for {
                              N: w1752 -> [_]
                              tunnel: w1751 -> [w1760]
                              tunnel: w1750 -> [w1757]
                              tunnel: w1749 -> [w1756]
                              i -> [w1761]
                              n696 = Multiply(x=2, y=w1761) -> (x*y=w1763:i32)
                              n697 = Increment(x=w1763) -> ()  [unwired: 1 out]
                              n698 = call "readbinary.vi"(7:w1757, "base path"=w1760, "file index"=w1763, "data column"="bcol") -> ("data"=w1759:ext[])  [unwired: 7 out]
                              n699 = call "writebinary.vi"(7:w1756, "base path"=w1760, "file index"=w1761, "data column"="bclt", "data"=w1759) -> ()  [unwired: 7 out]
                            }
                          }
                          frame #4 {
                            n700 = Array Size(array=w1771) -> (size(s)=w1770:i32)
                            n701 = Divide(x=w1770, y=2) -> (x/y=w1768:dbl)
                            n702 = for {
                              N: w1768 -> [_]
                              tunnel: w1767 -> [w1776]
                              tunnel: w1766 -> [w1773]
                              tunnel: w1765 -> [w1772]
                              i -> [w1777]
                              n703 = Multiply(x=2, y=w1777) -> (x*y=w1779:i32)
                              n704 = Increment(x=w1779) -> ()  [unwired: 1 out]
                              n705 = call "readbinary.vi"(7:w1773, "base path"=w1776, "file index"=w1779, "data column"="bdot") -> ("data"=w1775:ext[])  [unwired: 7 out]
                              n706 = call "writebinary.vi"(7:w1772, "base path"=w1776, "file index"=w1777, "data column"="bdtt", "data"=w1775) -> ()  [unwired: 7 out]
                            }
                          }
                          frame #5 {
                            n707 = Array Size(array=w1787) -> (size(s)=w1786:i32)
                            n708 = Divide(x=w1786, y=2) -> (x/y=w1784:dbl)
                            n709 = for {
                              N: w1784 -> [_]
                              tunnel: w1783 -> [w1792]
                              tunnel: w1782 -> [w1789]
                              tunnel: w1781 -> [w1788]
                              i -> [w1793]
                              n710 = Multiply(x=2, y=w1793) -> (x*y=w1795:i32)
                              n711 = Increment(x=w1795) -> ()  [unwired: 1 out]
                              n712 = call "readbinary.vi"(7:w1789, "base path"=w1792, "file index"=w1795, "data column"="indx") -> ("data"=w1791:ext[])  [unwired: 7 out]
                              n713 = call "writebinary.vi"(7:w1788, "base path"=w1792, "file index"=w1793, "data column"="indt", "data"=w1791) -> ()  [unwired: 7 out]
                            }
                          }
                          frame #6 {
                            n714 = Array Size(array=w1803) -> (size(s)=w1802:i32)
                            n715 = Divide(x=w1802, y=2) -> (x/y=w1800:dbl)
                            n716 = for {
                              N: w1800 -> [_]
                              tunnel: w1799 -> [w1808]
                              tunnel: w1798 -> [w1805]
                              tunnel: w1797 -> [w1804]
                              i -> [w1809]
                              n717 = Multiply(x=2, y=w1809) -> (x*y=w1811:i32)
                              n718 = Increment(x=w1811) -> ()  [unwired: 1 out]
                              n719 = call "readbinary.vi"(7:w1805, "base path"=w1808, "file index"=w1811, "data column"="time") -> ("data"=w1807:ext[])  [unwired: 7 out]
                              n720 = call "writebinary.vi"(7:w1804, "base path"=w1808, "file index"=w1809, "data column"="timt", "data"=w1807) -> ()  [unwired: 7 out]
                            }
                          }
                          frame #7 {
                            n721 = Array Size(array=w1824) -> (size(s)=w1827:i32)
                            n722 = Divide(x=w1827, y=2) -> (x/y=w1825:dbl)
                            n723 = for {
                              N: w1825 -> [_]
                              tunnel: w1813 -> [_]
                              tunnel: w1824 -> [w1836]
                              tunnel: w1823 -> [w1835]
                              tunnel: w1822 -> [w1832]
                              tunnel: [w1831] -> w1815 mode=indexing
                              tunnel: w1821 -> [w1830]
                              tunnel: [w1828] -> w1816 mode=indexing
                              i -> [w1838]
                              n724 = Multiply(x=2, y=w1838) -> (x*y=w1829:i32)
                              n725 = Index Array(array=w1836, index=w1829) -> (element=w1834:string)
                              n726 = Increment(x=w1829) -> (x+1=w1837:i32)
                              n727 = Index Array(array=w1836, index=w1837) -> (element=w1833:string)
                              n728 = case shown="1" w1835 {
                                tunnel: w1834 -> [w1840 w1846]
                                tunnel: w1833 -> [_ w1845]
                                tunnel: [w1840 w1843] -> w1831
                                tunnel: w1832 -> [_ w1844]
                                frame 0, Default {
                                }
                                frame 1 {
                                n729 = String Subset(string=w1846, length (rest)=w1844) -> (substring=w1842:string)  [unwired: 1 out]
                                n730 = String Subset(string=w1845, length (rest)=w1844) -> (substring=w1841:string)  [unwired: 1 out]
                                n731 = Concatenate Strings(w1841, w1842) -> (w1843:string)
                                }
                              }
                              n732 = Index Array(array=w1830, index=w1829) -> (element=w1828:path)
                            }
                            n733 = Build Path(base path=w1813, name or relative path="files2") -> (appended path=w1819:path)
                            n734 = call-poly <vilib>:"Write To Spreadsheet File.vi"("1D data"=w1815, "file path (dialog if empty)"=w1819) -> ()  [unwired: 4 in, 3 out]
                            n735 = Build Path(base path=w1813, name or relative path="paths2") -> (appended path=w1817:path)
                            n736 = Path To String(path=w1816) -> (string=w1814:string[])
                            n737 = call-poly <vilib>:"Write To Spreadsheet File.vi"("1D data"=w1814, "file path (dialog if empty)"=w1817) -> ()  [unwired: 4 in, 3 out]
                          }
                        }
                      }
                      frame 1 {
                        n738 = stacked-sequence {
                          seq-local: [w1854 _ _ _ _ _ _ _] -> [_ w1867 w1886 w1905 w1926 w1947 w1963 w1984]
                          seq-local: [w1852 _ _ _ _ _ _ _] -> [_ _ _ _ _ _ _ w1981]
                          tunnel: w1851 -> [w1858 w1863 w1882 w1901 w1922 w1943 w1959 w1973]
                          tunnel: w1850 -> [_ _ _ _ _ _ _ w1983]
                          tunnel: w1849 -> [_ _ _ _ _ _ _ w1982]
                          tunnel: w1848 -> [_ w1862 w1881 w1900 w1921 w1942 w1958 _]
                          tunnel: w1847 -> [_ w1861 w1880 w1899 w1920 w1941 w1957 _]
                          frame #0 {
                            w1856 = "%s"
                            n739 = Build Path(base path=w1858, name or relative path="files") -> (appended path=w1859:path)
                            n740 = call-poly <vilib>:"Read From Spreadsheet File.vi"("format (%s)"=w1856, "file path (dialog if empty)"=w1859) -> ("first row"=w1854:string[])  [unwired: 2 in, 7 out]
                            n741 = Build Path(base path=w1858, name or relative path="paths") -> (appended path=w1855:path)
                            n742 = call-poly <vilib>:"Read From Spreadsheet File.vi"("format (%s)"=w1856, "file path (dialog if empty)"=w1855) -> ("first row"=w1853:string[])  [unwired: 2 in, 7 out]
                            n743 = String To Path(string=w1853) -> (path=w1852:path[])
                          }
                          frame #1 {
                            n744 = Array Size(array=w1867) -> (size(s)=w1866:i32)
                            n745 = Divide(x=w1866, y=2) -> (x/y=w1864:dbl)
                            n746 = for {
                              N: w1864 -> [_]
                              tunnel: w1863 -> [w1873]
                              tunnel: w1862 -> [w1869]
                              tunnel: w1861 -> [w1868]
                              i -> [w1874]
                              w1876 = "dat1"
                              n747 = Multiply(x=2, y=w1874) -> (x*y=w1878:i32)
                              n748 = Increment(x=w1878) -> (x+1=w1877:i32)
                              n749 = call "readbinary.vi"(7:w1869, "base path"=w1873, "file index"=w1878, "data column"=w1876) -> ("data"=w1872:ext[])  [unwired: 7 out]
                              n750 = call "readbinary.vi"(7:w1869, "base path"=w1873, "file index"=w1877, "data column"=w1876) -> ("data"=w1871:ext[])  [unwired: 7 out]
                              n751 = Subtract(x=w1871, y=w1872) -> (x-y=w1875:ext[])
                              n752 = call "writebinary.vi"(7:w1868, "base path"=w1873, "file index"=w1874, "data column"="dt1t", "data"=w1875) -> ()  [unwired: 7 out]
                            }
                          }
                          frame #2 {
                            n753 = Array Size(array=w1886) -> (size(s)=w1885:i32)
                            n754 = Divide(x=w1885, y=2) -> (x/y=w1883:dbl)
                            n755 = for {
                              N: w1883 -> [_]
                              tunnel: w1882 -> [w1892]
                              tunnel: w1881 -> [w1888]
                              tunnel: w1880 -> [w1887]
                              i -> [w1893]
                              w1895 = "dat2"
                              n756 = Multiply(x=2, y=w1893) -> (x*y=w1897:i32)
                              n757 = Increment(x=w1897) -> (x+1=w1896:i32)
                              n758 = call "readbinary.vi"(7:w1888, "base path"=w1892, "file index"=w1897, "data column"=w1895) -> ("data"=w1890:ext[])  [unwired: 7 out]
                              n759 = call "readbinary.vi"(7:w1888, "base path"=w1892, "file index"=w1896, "data column"=w1895) -> ("data"=w1891:ext[])  [unwired: 7 out]
                              n760 = Subtract(x=w1891, y=w1890) -> (x-y=w1894:ext[])
                              n761 = call "writebinary.vi"(7:w1887, "base path"=w1892, "file index"=w1893, "data column"="dt2t", "data"=w1894) -> ()  [unwired: 7 out]
                            }
                          }
                          frame #3 {
                            n762 = Array Size(array=w1905) -> (size(s)=w1904:i32)
                            n763 = Divide(x=w1904, y=2) -> (x/y=w1902:dbl)
                            n764 = for {
                              N: w1902 -> [_]
                              tunnel: w1901 -> [w1914]
                              tunnel: w1900 -> [w1907]
                              tunnel: w1899 -> [w1906]
                              i -> [w1915]
                              w1916 = "bcol"
                              n765 = Multiply(x=2, y=w1915) -> (x*y=w1918:i32)
                              n766 = Increment(x=w1918) -> (x+1=w1917:i32)
                              n767 = call "readbinary.vi"(7:w1907, "base path"=w1914, "file index"=w1918, "data column"=w1916) -> ("data"=w1911:ext[])  [unwired: 7 out]
                              n768 = call "readbinary.vi"(7:w1907, "base path"=w1914, "file index"=w1917, "data column"=w1916) -> ("data"=w1910:ext[])  [unwired: 7 out]
                              n769 = Add(x=w1911, y=w1910) -> (x+y=w1913:ext[])
                              n770 = Divide(x=w1913, y=2) -> (x/y=w1909:ext[])
                              n771 = call "writebinary.vi"(7:w1906, "base path"=w1914, "file index"=w1915, "data column"="bclt", "data"=w1909) -> ()  [unwired: 7 out]
                            }
                          }
                          frame #4 {
                            n772 = Array Size(array=w1926) -> (size(s)=w1925:i32)
                            n773 = Divide(x=w1925, y=2) -> (x/y=w1923:dbl)
                            n774 = for {
                              N: w1923 -> [_]
                              tunnel: w1922 -> [w1935]
                              tunnel: w1921 -> [w1928]
                              tunnel: w1920 -> [w1927]
                              i -> [w1936]
                              w1937 = "bdot"
                              n775 = Multiply(x=2, y=w1936) -> (x*y=w1939:i32)
                              n776 = Increment(x=w1939) -> (x+1=w1938:i32)
                              n777 = call "readbinary.vi"(7:w1928, "base path"=w1935, "file index"=w1939, "data column"=w1937) -> ("data"=w1932:ext[])  [unwired: 7 out]
                              n778 = call "readbinary.vi"(7:w1928, "base path"=w1935, "file index"=w1938, "data column"=w1937) -> ("data"=w1931:ext[])  [unwired: 7 out]
                              n779 = Add(x=w1932, y=w1931) -> (x+y=w1934:ext[])
                              n780 = Divide(x=w1934, y=2) -> (x/y=w1930:ext[])
                              n781 = call "writebinary.vi"(7:w1927, "base path"=w1935, "file index"=w1936, "data column"="bdtt", "data"=w1930) -> ()  [unwired: 7 out]
                            }
                          }
                          frame #5 {
                            n782 = Array Size(array=w1947) -> (size(s)=w1946:i32)
                            n783 = Divide(x=w1946, y=2) -> (x/y=w1944:dbl)
                            n784 = for {
                              N: w1944 -> [_]
                              tunnel: w1943 -> [w1952]
                              tunnel: w1942 -> [w1949]
                              tunnel: w1941 -> [w1948]
                              i -> [w1953]
                              n785 = Multiply(x=2, y=w1953) -> (x*y=w1955:i32)
                              n786 = Increment(x=w1955) -> ()  [unwired: 1 out]
                              n787 = call "readbinary.vi"(7:w1949, "base path"=w1952, "file index"=w1955, "data column"="indx") -> ("data"=w1951:ext[])  [unwired: 7 out]
                              n788 = call "writebinary.vi"(7:w1948, "base path"=w1952, "file index"=w1953, "data column"="indt", "data"=w1951) -> ()  [unwired: 7 out]
                            }
                          }
                          frame #6 {
                            n789 = Array Size(array=w1963) -> (size(s)=w1962:i32)
                            n790 = Divide(x=w1962, y=2) -> (x/y=w1960:dbl)
                            n791 = for {
                              N: w1960 -> [_]
                              tunnel: w1959 -> [w1968]
                              tunnel: w1958 -> [w1965]
                              tunnel: w1957 -> [w1964]
                              i -> [w1969]
                              n792 = Multiply(x=2, y=w1969) -> (x*y=w1971:i32)
                              n793 = Increment(x=w1971) -> ()  [unwired: 1 out]
                              n794 = call "readbinary.vi"(7:w1965, "base path"=w1968, "file index"=w1971, "data column"="time") -> ("data"=w1967:ext[])  [unwired: 7 out]
                              n795 = call "writebinary.vi"(7:w1964, "base path"=w1968, "file index"=w1969, "data column"="timt", "data"=w1967) -> ()  [unwired: 7 out]
                            }
                          }
                          frame #7 {
                            n796 = Array Size(array=w1984) -> (size(s)=w1987:i32)
                            n797 = Divide(x=w1987, y=2) -> (x/y=w1985:dbl)
                            n798 = for {
                              N: w1985 -> [_]
                              tunnel: w1973 -> [_]
                              tunnel: w1984 -> [w1996]
                              tunnel: w1983 -> [w1995]
                              tunnel: w1982 -> [w1992]
                              tunnel: [w1991] -> w1975 mode=indexing
                              tunnel: w1981 -> [w1990]
                              tunnel: [w1988] -> w1976 mode=indexing
                              i -> [w1998]
                              n799 = Multiply(x=2, y=w1998) -> (x*y=w1989:i32)
                              n800 = Index Array(array=w1996, index=w1989) -> (element=w1994:string)
                              n801 = Increment(x=w1989) -> (x+1=w1997:i32)
                              n802 = Index Array(array=w1996, index=w1997) -> (element=w1993:string)
                              n803 = case shown="1" w1995 {
                                tunnel: w1994 -> [_ w2006]
                                tunnel: w1993 -> [w2000 w2005]
                                tunnel: [w2000 w2003] -> w1991
                                tunnel: w1992 -> [_ w2004]
                                frame 0, Default {
                                }
                                frame 1 {
                                n804 = String Subset(string=w2006, length (rest)=w2004) -> (substring=w2002:string)  [unwired: 1 out]
                                n805 = String Subset(string=w2005, length (rest)=w2004) -> (substring=w2001:string)  [unwired: 1 out]
                                n806 = Concatenate Strings(w2002, w2001) -> (w2003:string)
                                }
                              }
                              n807 = Index Array(array=w1990, index=w1989) -> (element=w1988:path)
                            }
                            n808 = Build Path(base path=w1973, name or relative path="files2") -> (appended path=w1979:path)
                            n809 = call-poly <vilib>:"Write To Spreadsheet File.vi"("1D data"=w1975, "file path (dialog if empty)"=w1979) -> ()  [unwired: 4 in, 3 out]
                            n810 = Build Path(base path=w1973, name or relative path="paths2") -> (appended path=w1977:path)
                            n811 = Path To String(path=w1976) -> (string=w1974:string[])
                            n812 = call-poly <vilib>:"Write To Spreadsheet File.vi"("1D data"=w1974, "file path (dialog if empty)"=w1977) -> ()  [unwired: 4 in, 3 out]
                          }
                        }
                      }
                      frame 3 {
                        n813 = stacked-sequence {
                          seq-local: [w2014 _ _ _ _ _ _ _] -> [_ w2027 w2046 w2065 w2082 w2099 w2115 w2136]
                          seq-local: [w2012 _ _ _ _ _ _ _] -> [_ _ _ _ _ _ _ w2133]
                          tunnel: w2011 -> [w2018 w2023 w2042 w2061 w2078 w2095 w2111 w2125]
                          tunnel: w2010 -> [_ _ _ _ _ _ _ w2135]
                          tunnel: w2009 -> [_ _ _ _ _ _ _ w2134]
                          tunnel: w2008 -> [_ w2022 w2041 w2060 w2077 w2094 w2110 _]
                          tunnel: w2007 -> [_ w2021 w2040 w2059 w2076 w2093 w2109 _]
                          frame #0 {
                            w2016 = "%s"
                            n814 = Build Path(base path=w2018, name or relative path="files") -> (appended path=w2019:path)
                            n815 = call-poly <vilib>:"Read From Spreadsheet File.vi"("format (%s)"=w2016, "file path (dialog if empty)"=w2019) -> ("first row"=w2014:string[])  [unwired: 2 in, 7 out]
                            n816 = Build Path(base path=w2018, name or relative path="paths") -> (appended path=w2015:path)
                            n817 = call-poly <vilib>:"Read From Spreadsheet File.vi"("format (%s)"=w2016, "file path (dialog if empty)"=w2015) -> ("first row"=w2013:string[])  [unwired: 2 in, 7 out]
                            n818 = String To Path(string=w2013) -> (path=w2012:path[])
                          }
                          frame #1 {
                            n819 = Array Size(array=w2027) -> (size(s)=w2026:i32)
                            n820 = Divide(x=w2026, y=2) -> (x/y=w2024:dbl)
                            n821 = for {
                              N: w2024 -> [_]
                              tunnel: w2023 -> [w2033]
                              tunnel: w2022 -> [w2029]
                              tunnel: w2021 -> [w2028]
                              i -> [w2034]
                              w2036 = "dat1"
                              n822 = Multiply(x=2, y=w2034) -> (x*y=w2038:i32)
                              n823 = Increment(x=w2038) -> (x+1=w2037:i32)
                              n824 = call "readbinary.vi"(7:w2029, "base path"=w2033, "file index"=w2038, "data column"=w2036) -> ("data"=w2032:ext[])  [unwired: 7 out]
                              n825 = call "readbinary.vi"(7:w2029, "base path"=w2033, "file index"=w2037, "data column"=w2036) -> ("data"=w2031:ext[])  [unwired: 7 out]
                              n826 = Subtract(x=w2031, y=w2032) -> (x-y=w2035:ext[])
                              n827 = call "writebinary.vi"(7:w2028, "base path"=w2033, "file index"=w2034, "data column"="dt1t", "data"=w2035) -> ()  [unwired: 7 out]
                            }
                          }
                          frame #2 {
                            n828 = Array Size(array=w2046) -> (size(s)=w2045:i32)
                            n829 = Divide(x=w2045, y=2) -> (x/y=w2043:dbl)
                            n830 = for {
                              N: w2043 -> [_]
                              tunnel: w2042 -> [w2052]
                              tunnel: w2041 -> [w2048]
                              tunnel: w2040 -> [w2047]
                              i -> [w2053]
                              w2055 = "dat2"
                              n831 = Multiply(x=2, y=w2053) -> (x*y=w2057:i32)
                              n832 = Increment(x=w2057) -> (x+1=w2056:i32)
                              n833 = call "readbinary.vi"(7:w2048, "base path"=w2052, "file index"=w2057, "data column"=w2055) -> ("data"=w2050:ext[])  [unwired: 7 out]
                              n834 = call "readbinary.vi"(7:w2048, "base path"=w2052, "file index"=w2056, "data column"=w2055) -> ("data"=w2051:ext[])  [unwired: 7 out]
                              n835 = Subtract(x=w2051, y=w2050) -> (x-y=w2054:ext[])
                              n836 = call "writebinary.vi"(7:w2047, "base path"=w2052, "file index"=w2053, "data column"="dt2t", "data"=w2054) -> ()  [unwired: 7 out]
                            }
                          }
                          frame #3 {
                            n837 = Array Size(array=w2065) -> (size(s)=w2064:i32)
                            n838 = Divide(x=w2064, y=2) -> (x/y=w2062:dbl)
                            n839 = for {
                              N: w2062 -> [_]
                              tunnel: w2061 -> [w2071]
                              tunnel: w2060 -> [w2067]
                              tunnel: w2059 -> [w2066]
                              i -> [w2072]
                              n840 = Multiply(x=2, y=w2072) -> (x*y=w2074:i32)
                              n841 = Increment(x=w2074) -> (x+1=w2073:i32)
                              n842 = call "readbinary.vi"(7:w2067, "base path"=w2071, "file index"=w2073, "data column"="bcol") -> ("data"=w2070:ext[])  [unwired: 7 out]
                              n843 = call "writebinary.vi"(7:w2066, "base path"=w2071, "file index"=w2072, "data column"="bclt", "data"=w2070) -> ()  [unwired: 7 out]
                            }
                          }
